vi "Multiplexer_Ch_No.vi"(0 "Channel Number":i16) -> (1 "Multiplexer Ch No":i16, 2 "ADC Ch No":i16)   [LabVIEW 2012]
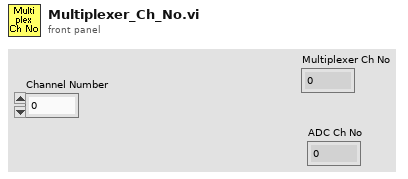
[diagram p1: front panel]
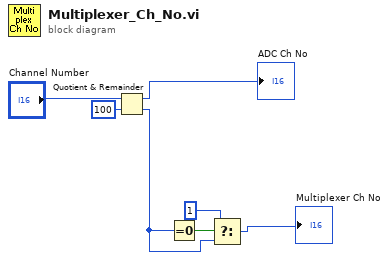
[diagram p0: block diagram]
diagram:
  n1 = Quotient & Remainder(x="Channel Number", y=i16 100) -> (x-y*floor(x/y)=→"ADC Ch No":i16, floor(x/y)=w3:i16)
  n2 = Equal To 0?(x=w3) -> (x = 0?=w4:bool)
  n3 = Select(t=i16 1, s=w4, f=w3) -> (s? t:f=→"Multiplexer Ch No":i16)
